vi "reboot.vi"(8 "error in (no error)":errorcluster, 10 "SendTo":string, 11 "service":refnum<class "IcmMessageService.lvclass">) -> (0 "error out":errorcluster)   [LabVIEW 2017]
uses:
  <vilib>/addons/InsightCM/MessageBus/MessageService/IcmMessageService.lvclass
  <vilib>/addons/InsightCM/MessageBus/Base/controls/Message.ctl
  <vilib>/addons/InsightCM/MessageBus/Base/controls/MessageHeader.ctl
  <vilib>/addons/InsightCM/MessageBus/Base/controls/KeyValuePair.ctl
panel:
  out "data string":string
  out "response":T1
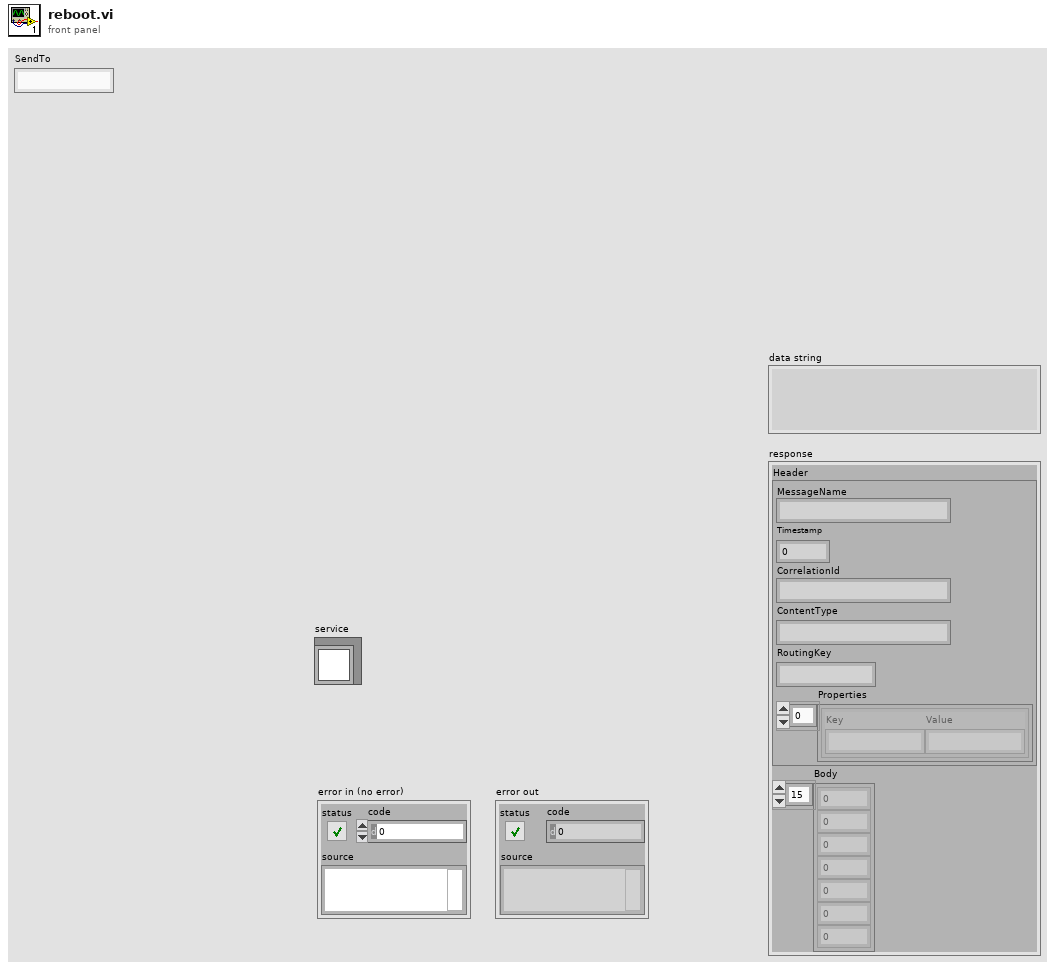
[diagram p1: front panel]
types:
  T1 = typedef "Message.ctl" = cluster{"Header":T2, "Body":u8[]}
  T2 = typedef "MessageHeader.ctl" = cluster{"MessageName":string, "Timestamp":i64, "CorrelationId":string, "ContentType":string, "RoutingKey":string, "Properties":T3[]}
  T3 = typedef "KeyValuePair.ctl" = cluster{"Key":string, "Value":string}
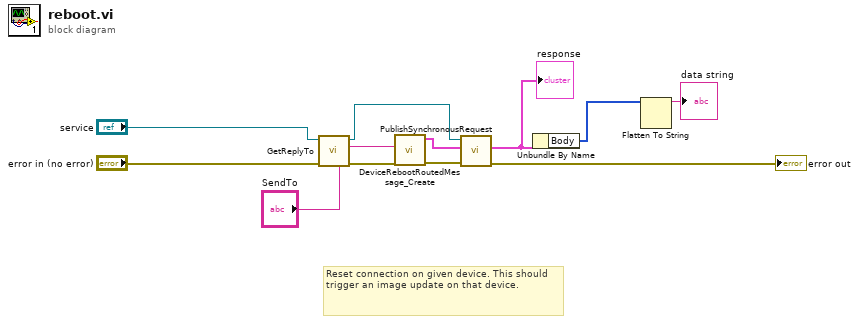
[diagram p0: block diagram]
diagram:
  # "Reset connection on given device. This should trigger an image update on that device."
  n1 = call <vilib>:"GetReplyTo.vi"("error in (no error)"="error in (no error)", "service in"="service") -> ("error out"=w4:errorcluster, "service out"=w9:refnum<class "IcmMessageService.lvclass">)  [unwired: 7 in, 1 out]
  n2 = call <vilib>:"DeviceRebootRoutedMessage_Create.vi"("error in (no error)"=w4, "SendTo"="SendTo") -> ("error out"=w3:errorcluster, "Message"=w1:T1)  [unwired: 8 in]
  n3 = call <vilib>:"PublishSynchronousRequest.vi"("error in (no error)"=w3, "request"=w1, "service in"=w9) -> ("error out"=→"error out":errorcluster, "response"=w7:T1)  [unwired: 6 in, 1 out]
  "response" <- w7
  n4 = Unbundle By Name(w7) -> ("Body"=w6:u8[])
  n5 = Flatten To String(anything=w6) -> (data string=→"data string":string)  [unwired: 3 in, 2 out]
